vi "Finish.vi"   [LabVIEW 2016]
doc: "This VI is called just before exiting. It is expected to close I/O refnum, save collected data, etc."
uses:
  <vilib>/Rock Robotics/WPI/Utilities/WPI_GetSetVariantRefNum.vi
types:
  T1 = typedef "WPI_JoystickDevRef.ctl" = cluster{"Device":T2}
  T2 = typedef "WPI_JoystickDeviceEnum.ctl" = enum16{"USB 0", "USB 1", "USB 2", "USB 3", "USB 4", "USB 5"}
  T3 = typedef "WPI_RobotDriveDevRef.ctl" = cluster{"DevStatus":errorcluster, "Motors[]":T4[], "Square Inputs":bool, "Max Output":dbl}
  T4 = typedef "WPI_MotorControlDeviceRef.ctl" = cluster{"DeviceStatus":errorcluster, "Type":T5, "PWM":cluster{"PWM Channel":T6, "DeadBand":T7}, "CAN":cluster{"Device Number":u8, "SetOutput VI Ref":variant, "GetOutput VI Ref":variant, "Enable VI Ref":variant, "Disable VI Ref":variant, "Data":variant}, "Invert":bool}
  T5 = typedef "WPI_MotorControlType.ctl" = enum16{"PWM", "CAN"}
  T6 = typedef "FPGA_DIOPWMChannel.ctl" = enum8{"PWM 0", "PWM 1", "PWM 2", "PWM 3", "PWM 4", "PWM 5", "PWM 6", "PWM 7", "PWM 8", "PWM 9", "PWM MXP 0", "PWM MXP 1", "PWM MXP 2", "PWM MXP 3", "PWM MXP 4", "PWM MXP 5", "PWM MXP 6", "PWM MXP 7", "PWM MXP 8", "PWM MXP 9", "Invalid"}
  T7 = typedef "WPI_PWMDeadband.ctl" = cluster{"Name":string, "maxPositivePwm":i32, "minPositivePwm":i32, "centerPwm":i32, "maxNegativePwm":i32, "minNegativePwm":i32, "angularRange":u16}
  T8 = typedef "WPI_DigitalInputDevRef.ctl" = cluster{"DevStatus":errorcluster, "DIO Channel":T9}
  T9 = typedef "FPGA_DIOChannel.ctl" = enum8{"DIO 0", "DIO 1", "DIO 2", "DIO 3", "DIO 4", "DIO 5", "DIO 6", "DIO 7", "DIO 8", "DIO 9", "DIO MXP 0", "DIO MXP 1", "DIO MXP 2", "DIO MXP 3", "DIO MXP 4", "DIO MXP 5", "DIO MXP 6", "DIO MXP 7", "DIO MXP 8", "DIO MXP 9", "DIO MXP 10", "DIO MXP 11", "DIO MXP 12", "DIO MXP 13", "DIO MXP 14", "DIO MXP 15", "SPI Port CS1", "SPI Port CS2", "SPI Port CS3", "SPI Port MISO", "SPI Port MOSI", "Invalid"}
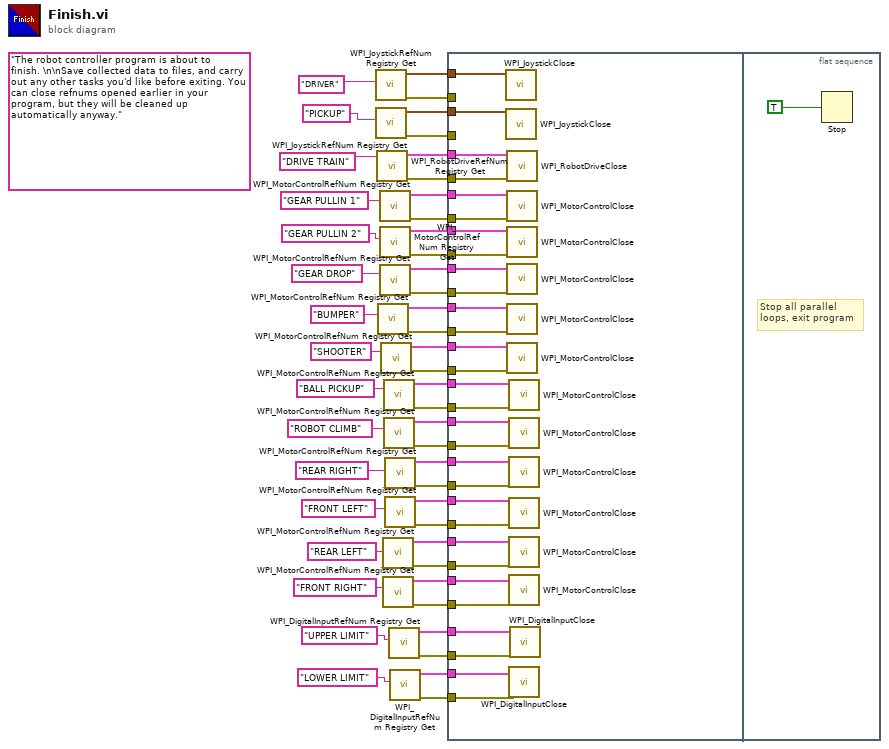
[diagram p0: block diagram]
diagram:
  (unwired) "The robot controller program is about to finish. \n\nSave collected data to files, and carry out any other tasks you'd like before exiting. You can close refnums opened earlier in your program, but they will be cleaned up automatically anyway."
  n1 = call <vilib>:"WPI_JoystickRefNum Registry Get.vi"("refnum name"="DRIVER") -> ("error out"=w22:errorcluster, "JoystickDevRef"=w45:T1)  [unwired: 1 in, 8 out]
  n2 = call <vilib>:"WPI_JoystickRefNum Registry Get.vi"("refnum name"="PICKUP") -> ("error out"=w20:errorcluster, "JoystickDevRef"=w21:T1)  [unwired: 1 in, 8 out]
  n3 = call <vilib>:"WPI_RobotDriveRefNum Registry Get.vi"("refnum name"="DRIVE TRAIN") -> ("error out"=w19:errorcluster, "RobotDriveDevRef"=w46:T3)  [unwired: 1 in, 8 out]
  n4 = call <vilib>:"WPI_MotorControlRefNum Registry Get.vi"("refnum name"="BUMPER") -> ("error out"=w29:errorcluster, "MotorControlDevRef"=w30:T4)  [unwired: 9 in]
  n5 = call <vilib>:"WPI_MotorControlRefNum Registry Get.vi"("refnum name"="GEAR PULLIN 1") -> ("error out"=w35:errorcluster, "MotorControlDevRef"=w36:T4)  [unwired: 9 in]
  n6 = call <vilib>:"WPI_MotorControlRefNum Registry Get.vi"("refnum name"="GEAR PULLIN 2") -> ("error out"=w33:errorcluster, "MotorControlDevRef"=w34:T4)  [unwired: 9 in]
  n7 = call <vilib>:"WPI_MotorControlRefNum Registry Get.vi"("refnum name"="GEAR DROP") -> ("error out"=w31:errorcluster, "MotorControlDevRef"=w32:T4)  [unwired: 9 in]
  n8 = call <vilib>:"WPI_MotorControlRefNum Registry Get.vi"("refnum name"="SHOOTER") -> ("error out"=w27:errorcluster, "MotorControlDevRef"=w28:T4)  [unwired: 9 in]
  n9 = call <vilib>:"WPI_MotorControlRefNum Registry Get.vi"("refnum name"="REAR LEFT") -> ("error out"=w13:errorcluster, "MotorControlDevRef"=w14:T4)  [unwired: 9 in]
  n10 = call <vilib>:"WPI_MotorControlRefNum Registry Get.vi"("refnum name"="FRONT RIGHT") -> ("error out"=w11:errorcluster, "MotorControlDevRef"=w12:T4)  [unwired: 9 in]
  n11 = call <vilib>:"WPI_MotorControlRefNum Registry Get.vi"("refnum name"="BALL PICKUP") -> ("error out"=w25:errorcluster, "MotorControlDevRef"=w26:T4)  [unwired: 9 in]
  n12 = call <vilib>:"WPI_MotorControlRefNum Registry Get.vi"("refnum name"="ROBOT CLIMB") -> ("error out"=w23:errorcluster, "MotorControlDevRef"=w24:T4)  [unwired: 9 in]
  n13 = call <vilib>:"WPI_MotorControlRefNum Registry Get.vi"("refnum name"="REAR RIGHT") -> ("error out"=w17:errorcluster, "MotorControlDevRef"=w18:T4)  [unwired: 9 in]
  n14 = call <vilib>:"WPI_MotorControlRefNum Registry Get.vi"("refnum name"="FRONT LEFT") -> ("error out"=w15:errorcluster, "MotorControlDevRef"=w16:T4)  [unwired: 9 in]
  n15 = call <vilib>:"WPI_DigitalInputRefNum Registry Get.vi"("refnum name"="UPPER LIMIT") -> ("error out"=w2:errorcluster, "DigitalInputDevRef"=w3:T8)  [unwired: 9 in]
  n16 = call <vilib>:"WPI_DigitalInputRefNum Registry Get.vi"("refnum name"="LOWER LIMIT") -> ("error out"=w1:errorcluster, "DigitalInputDevRef"=w4:T8)  [unwired: 9 in]
  n17 = flat-sequence {
    tunnel: w46 -> [w78]
    tunnel: w45 -> [w77]
    tunnel: w36 -> [w74]
    tunnel: w35 -> [w73]
    tunnel: w34 -> [w72]
    tunnel: w33 -> [w71]
    tunnel: w32 -> [w70]
    tunnel: w31 -> [w69]
    tunnel: w30 -> [w68]
    tunnel: w29 -> [w67]
    tunnel: w28 -> [w66]
    tunnel: w27 -> [w65]
    tunnel: w26 -> [w64]
    tunnel: w25 -> [w63]
    tunnel: w24 -> [w62]
    tunnel: w23 -> [w61]
    tunnel: w22 -> [_]
    tunnel: w21 -> [w76]
    tunnel: w20 -> [_]
    tunnel: w19 -> [w75]
    tunnel: w18 -> [w60]
    tunnel: w17 -> [w59]
    tunnel: w16 -> [w58]
    tunnel: w15 -> [w57]
    tunnel: w14 -> [w56]
    tunnel: w13 -> [w55]
    tunnel: w12 -> [w54]
    tunnel: w11 -> [w53]
    tunnel: w4 -> [w52]
    tunnel: w3 -> [w51]
    tunnel: w2 -> [w50]
    tunnel: w1 -> [w49]
    frame #0 {
      n18 = call <vilib>:"WPI_JoystickClose.vi"("JoystickDevRef"=w77) -> ()  [unwired: 11 out]
      n19 = call <vilib>:"WPI_JoystickClose.vi"("JoystickDevRef"=w76) -> ()  [unwired: 11 out]
      n20 = call <vilib>:"WPI_RobotDriveClose.vi"("error in (no error)"=w75, "RobotDriveDevRef"=w78) -> ()  [unwired: 10 out]
      n21 = call <vilib>:"WPI_MotorControlClose.vi"("error in"=w73, "MotorControlDevRef"=w74) -> ()  [unwired: 9 in, 1 out]
      n22 = call <vilib>:"WPI_MotorControlClose.vi"("error in"=w71, "MotorControlDevRef"=w72) -> ()  [unwired: 9 in, 1 out]
      n23 = call <vilib>:"WPI_MotorControlClose.vi"("error in"=w69, "MotorControlDevRef"=w70) -> ()  [unwired: 9 in, 1 out]
      n24 = call <vilib>:"WPI_MotorControlClose.vi"("error in"=w67, "MotorControlDevRef"=w68) -> ()  [unwired: 9 in, 1 out]
      n25 = call <vilib>:"WPI_MotorControlClose.vi"("error in"=w65, "MotorControlDevRef"=w66) -> ()  [unwired: 9 in, 1 out]
      n26 = call <vilib>:"WPI_MotorControlClose.vi"("error in"=w63, "MotorControlDevRef"=w64) -> ()  [unwired: 9 in, 1 out]
      n27 = call <vilib>:"WPI_MotorControlClose.vi"("error in"=w61, "MotorControlDevRef"=w62) -> ()  [unwired: 9 in, 1 out]
      n28 = call <vilib>:"WPI_MotorControlClose.vi"("error in"=w59, "MotorControlDevRef"=w60) -> ()  [unwired: 9 in, 1 out]
      n29 = call <vilib>:"WPI_MotorControlClose.vi"("error in"=w57, "MotorControlDevRef"=w58) -> ()  [unwired: 9 in, 1 out]
      n30 = call <vilib>:"WPI_MotorControlClose.vi"("error in"=w55, "MotorControlDevRef"=w56) -> ()  [unwired: 9 in, 1 out]
      n31 = call <vilib>:"WPI_MotorControlClose.vi"("error in"=w53, "MotorControlDevRef"=w54) -> ()  [unwired: 9 in, 1 out]
      n32 = call <vilib>:"WPI_DigitalInputClose.vi"("error in (no error)"=w49, "DigitalInputDevRef"=w52) -> ()  [unwired: 9 in, 1 out]
      n33 = call <vilib>:"WPI_DigitalInputClose.vi"("error in (no error)"=w50, "DigitalInputDevRef"=w51) -> ()  [unwired: 9 in, 1 out]
    }
    frame #1 {
      # "Stop all parallel\nloops, exit program"
      n34 = Stop(stop? (T)=TRUE ("Quit")) -> ()
    }
  }
